vi "Set Car Wash Started Event.vi"(7 "Name":string, 8 "error in (no error)":errorcluster, 10 "Format":string, 11 "Wash Options":string[](array[string])) -> (0 "error out":errorcluster, 3 "Car Wash Started out":refnum<class "Car Wash Started.lvclass">)   [LabVIEW 2016, in "CLD Exam - Car Wash.lvlib" / "Car Wash Started.lvclass"]
uses:
  Car Wash Started.lvclass
  D:/Repos/Stream/software/Mediator/Classes/Message Interface/Message Interface.lvclass
  Car Wash Started.lvclass/Car Wash Started.ctl
  Mediator/Classes/Message Interface/Message Interface.lvclass
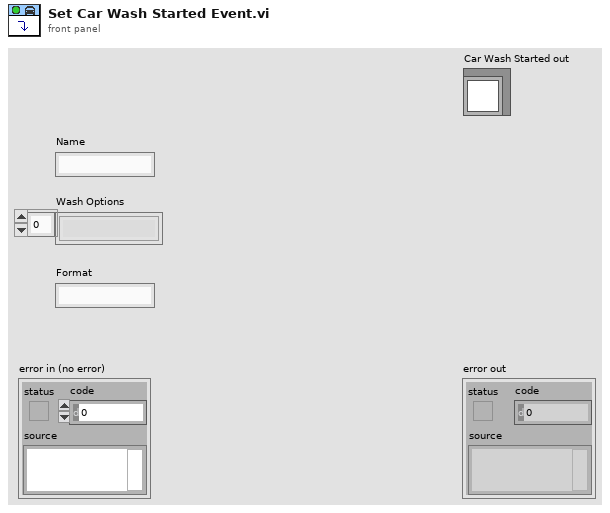
[diagram p1: front panel]
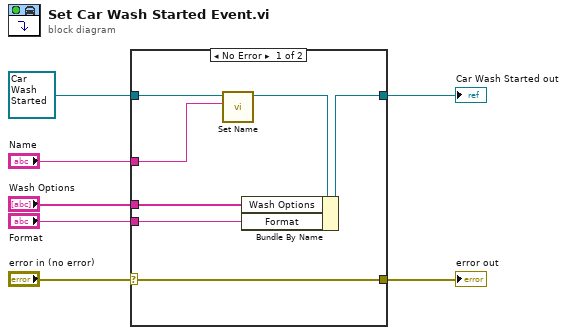
[diagram p0: block diagram]
diagram:
  n1 = case shown="No Error" "error in (no error)" {
    selector: "error in (no error)" -> [w14 w16]
    tunnel: [w14 w16] -> w6
    tunnel: [w10 w15] -> w4
    tunnel: refnum<class "Car Wash Started.lvclass"> refnum ("Car Wash Started in") -> [w13 w15]
    tunnel: "Name" -> [w12 _]
    tunnel: "Wash Options" -> [w9 _]
    tunnel: "Format" -> [w8 _]
    frame No Error {
      n2 = call "Set Name.vi"("Name"=w12, "Message Interface in"=w13) -> ("Message Interface out"=w11:refnum<class "Car Wash Started.lvclass">)  [unwired: 8 in, 1 out]
      n3 = Bundle By Name(cluster=w11, "Wash Options"=w9, "Format"=w8) -> (w10:refnum<class "Car Wash Started.lvclass">)
    }
    frame Error {
    }
  }
  "error out" <- w6
  "Car Wash Started out" <- w4
